vi "subDisplayMessage.vi"(5 "Second Button Name":string, 7 "Button Name":string, 8 "error in (no error)":errorcluster, 9 "Enable Message":bool, 10 "Show 'Cancel' Button":bool, 11 "Message to Display":string) -> (0 "error out":errorcluster, 2 "OK?":bool)   [LabVIEW 2020]
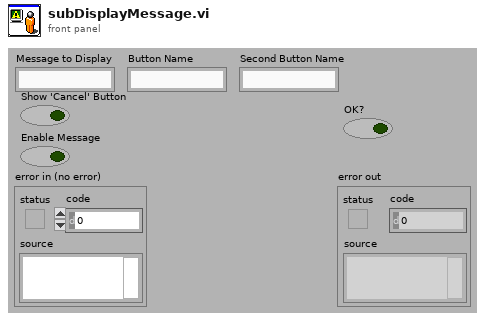
[diagram p1: front panel]
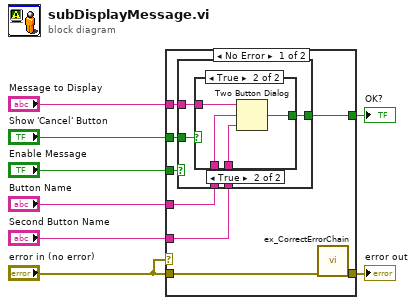
[diagram p0: block diagram]
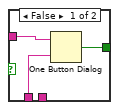
[diagram p3: hidden frame]
diagram:
  n1 = case shown="No Error" "error in (no error)" {
    tunnel: "Button Name" -> [w16 _]
    tunnel: "Second Button Name" -> [w15 _]
    tunnel: "Enable Message" -> [w14 _]
    tunnel: "Show 'Cancel' Button" -> [w13 _]
    tunnel: [w12 _] -> w4
    tunnel: "Message to Display" -> [w11 _]
    tunnel: "error in (no error)" -> [w10 w30]
    tunnel: [w9 w30] -> w2
    frame No Error {
      n2 = case shown="True" w14 {
        selector: w14 -> [w17 _]
        tunnel: w11 -> [_ w22]
        tunnel: [w17 w21] -> w12
        tunnel: w13 -> [_ w20]
        tunnel: w15 -> [_ w19]
        tunnel: w16 -> [_ w18]
        frame False {
        }
        frame True {
          n3 = case shown="True" w20 {
            tunnel: w22 -> [w25 w29]
            tunnel: [w24 w28] -> w21
            tunnel: w19 -> [_ w26]
            tunnel: w18 -> [w23 w27]
            frame False {
              n4 = One Button Dialog(message=w25, button name ("OK")=w23) -> (true=w24:bool)
            }
            frame True {
              n5 = Two Button Dialog(message=w29, 1:w26, 2:w27) -> (T button?=w28:bool)
            }
          }
        }
      }
      n6 = call "ex_CorrectErrorChain.vi"("error in (no error)"=w10) -> ("error out"=w9:errorcluster)  [unwired: 10 in]
    }
    frame Error {
    }
  }
  "OK?" <- w4
  "error out" <- w2
